vi "GlobalVariables.vi"() -> ()   [LabVIEW 2021]
panel:
  out "Image":T1(plugin-control)
  in  "AbortAutoFocus":bool
  in  "StopJoyStick":bool
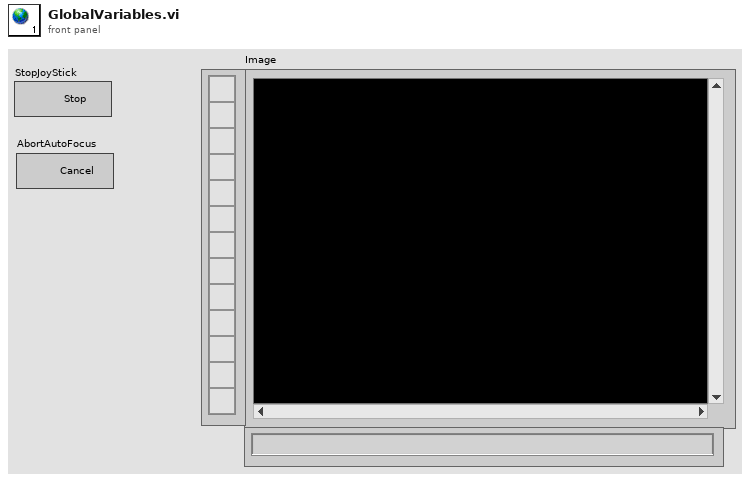
[diagram p1: front panel]
types:
  T1 = typedef "IMAQ Image.ctl" = refnum<image>
diagram:
